vi "about_v1.0.vi"() -> ()   [LabVIEW 2025]
doc: "Use this template to build a producer/consumer design pattern with events to produce queue items. Use this design pattern instead of the User Interface Event Handler pattern for user interfaces when you want to execute code asynchronously in response to an event without slowing the user interface responsiveness."
uses:
  controls/hyperlink.ctl
  controls/linkedin.ctl
  controls/fb.ctl
  controls/youtube.ctl
  controls/insta.ctl
  controls/x.ctl
  <vilib>/Platform/browser.llb/Open URL in Default Browser (string).vi
panel:
  in  "x":T1
  in  "insta":T2
  in  "youtube":T3
  in  "facebook":T4
  in  "linkedin":T5
  in  "producer_exit":bool
  in  "hyperlink":T6
  # "Fresh was founded in 2007 with the vision of pairing design and technology to drive innovation in the emerging digital economy.\n\nJeff Dance and Steve Hulet, our co-founders, imagined multi-disciplinary teams coming together to solve challenges for today and tomorrow, leveraging the best talent and technology in the process.\n\nAs Fresh grows, we remain committed to integrated teams, truly collaborative teamwork, and honing the combination of creative and technical consulting."
  # "Contact Us"
  # "HQ"
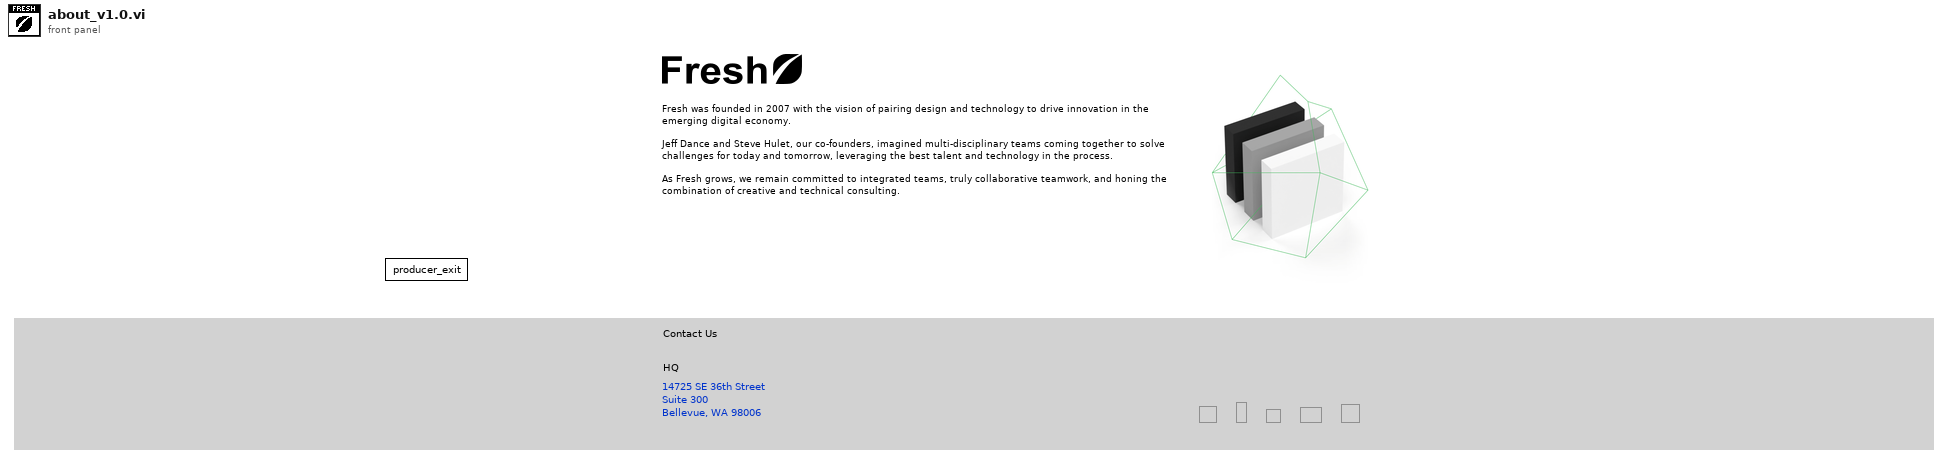
[diagram p1: front panel]
types:
  T1 = typedef "x.ctl" = bool
  T2 = typedef "insta.ctl" = bool
  T3 = typedef "youtube.ctl" = bool
  T4 = typedef "fb.ctl" = bool
  T5 = typedef "linkedin.ctl" = bool
  T6 = typedef "hyperlink.ctl" = bool
  T7 = enum32{"Invalid", "Standard", "Closed", "Hidden", "Minimized", "Maximized"}
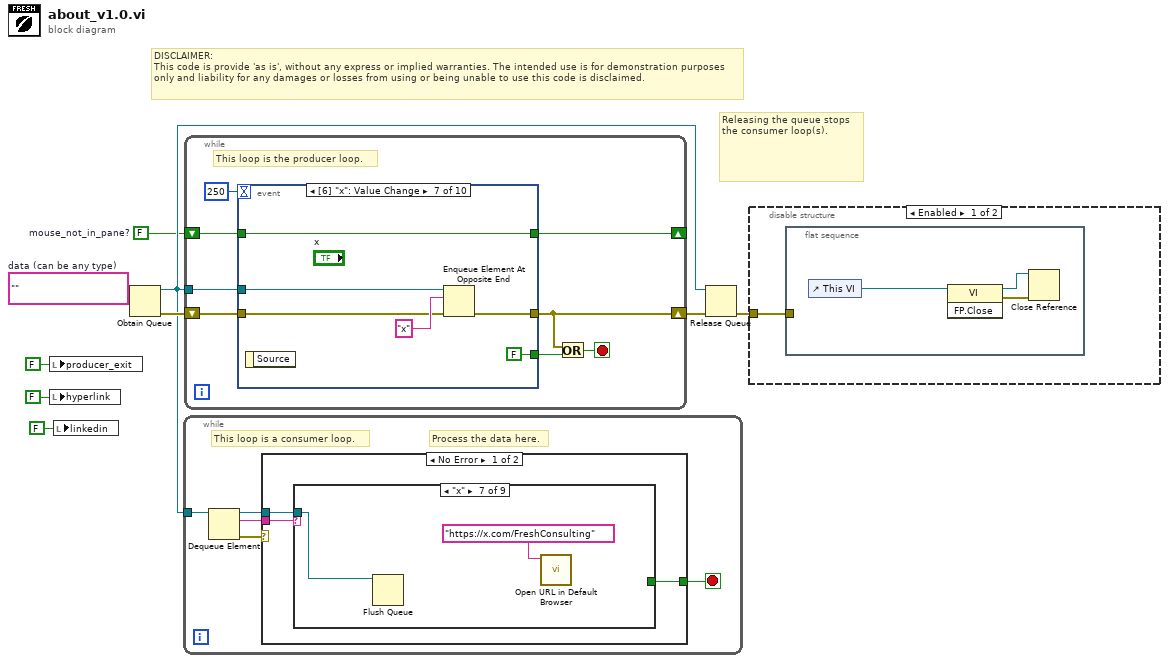
[diagram p0: block diagram]
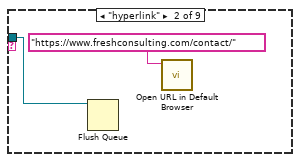
[diagram p4: hidden frame]
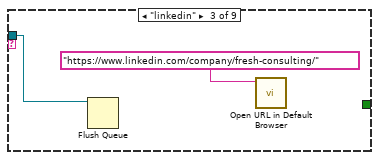
[diagram p5: hidden frame]
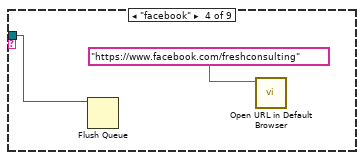
[diagram p6: hidden frame]
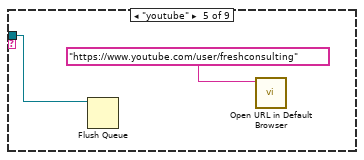
[diagram p7: hidden frame]
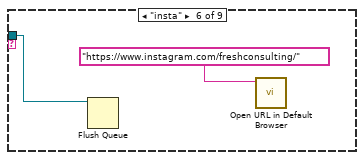
[diagram p8: hidden frame]
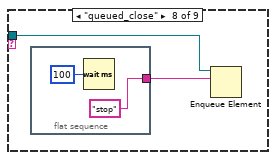
[diagram p9: hidden frame]
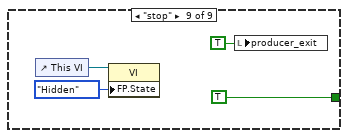
[diagram p10: hidden frame]
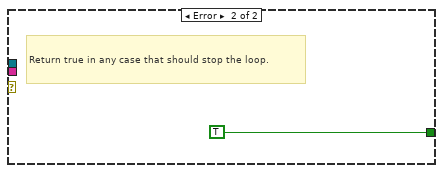
[diagram p11: hidden frame]
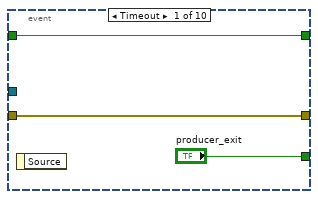
[diagram p12: hidden frame]
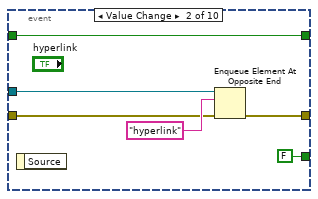
[diagram p13: hidden frame]
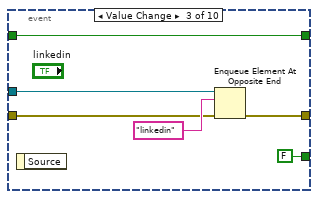
[diagram p14: hidden frame]
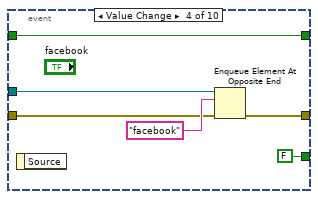
[diagram p15: hidden frame]
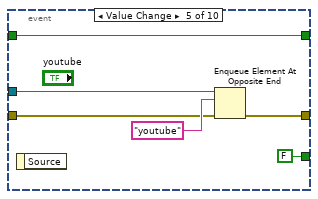
[diagram p16: hidden frame]
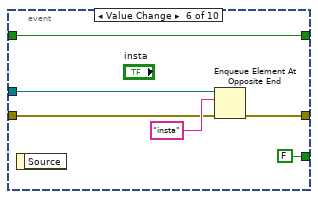
[diagram p17: hidden frame]
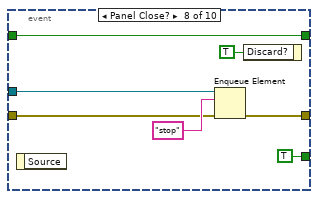
[diagram p18: hidden frame]
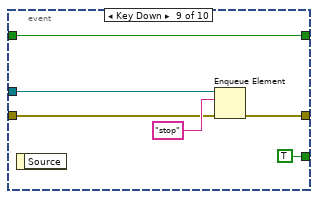
[diagram p19: hidden frame]
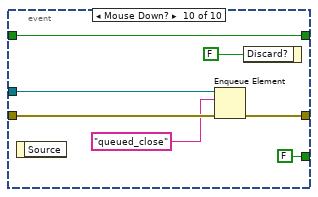
[diagram p20: hidden frame]
diagram:
  w4 = FALSE  # mouse_not_in_pane?
  w7 = ""  # data (can be any type)
  # "DISCLAIMER:\nThis code is provide 'as is', without any express or implied warranties. The intended use is for demonstration purposes only and liability for any damages or losses from using or being unable to use this code is disclaimed."
  # "Releasing the queue stops the consumer loop(s)."
  n1 = local write "producer_exit"(FALSE ("producer_exit")) -> ()
  n2 = local write "hyperlink"(T6 FALSE ("hyperlink")) -> ()
  n3 = local write "linkedin"(T5 FALSE ("linkedin")) -> ()
  n4 = Obtain Queue(element data type=w7) -> (queue out=w6:refnum<queue>, error out=w9:errorcluster)  [unwired: 4 in, 1 out]
  n5 = while {
    tunnel: w6 -> [w14]
    stop <- w11 stop-if-true
    # "Process the data here."
    # "This loop is a consumer loop."
    n6 = Dequeue Element(queue=w14) -> (queue out=w10:refnum<queue>, element=w12:string, error out=w13:errorcluster)  [unwired: 2 in, 1 out]
    n7 = case shown="No Error" w13 {
      tunnel: w12 -> [w17 _]
      tunnel: [w16 TRUE] -> w11
      tunnel: w10 -> [w15 _]
      frame No Error {
        n8 = case shown="\"x\"" w17 {
          tunnel: [_ _ _ _ _ _ _ _ TRUE] -> w16
          tunnel: w15 -> [_ w18 w20 w22 w24 w26 w28 w31 _]
          frame Default {
          }
          frame "hyperlink" {
            n9 = Flush Queue(queue=w18) -> ()  [unwired: 1 in, 3 out]
            n10 = call-poly <vilib>:"Open URL in Default Browser.vi"("URL"="https://www.freshconsulting.com/contact/") -> ()  [unwired: 5 in, 2 out]
          }
          frame "linkedin" {
            n11 = Flush Queue(queue=w20) -> ()  [unwired: 1 in, 3 out]
            n12 = call-poly <vilib>:"Open URL in Default Browser.vi"("URL"="https://www.linkedin.com/company/fresh-consulting/") -> ()  [unwired: 5 in, 2 out]
          }
          frame "facebook" {
            n13 = Flush Queue(queue=w22) -> ()  [unwired: 1 in, 3 out]
            n14 = call-poly <vilib>:"Open URL in Default Browser.vi"("URL"="https://www.facebook.com/freshconsulting") -> ()  [unwired: 5 in, 2 out]
          }
          frame "youtube" {
            n15 = Flush Queue(queue=w24) -> ()  [unwired: 1 in, 3 out]
            n16 = call-poly <vilib>:"Open URL in Default Browser.vi"("URL"="https://www.youtube.com/user/freshconsulting") -> ()  [unwired: 5 in, 2 out]
          }
          frame "insta" {
            n17 = Flush Queue(queue=w26) -> ()  [unwired: 1 in, 3 out]
            n18 = call-poly <vilib>:"Open URL in Default Browser.vi"("URL"="https://www.instagram.com/freshconsulting/") -> ()  [unwired: 5 in, 2 out]
          }
          frame "x" {
            n19 = Flush Queue(queue=w28) -> ()  [unwired: 1 in, 3 out]
            n20 = call-poly <vilib>:"Open URL in Default Browser.vi"("URL"="https://x.com/FreshConsulting") -> ()  [unwired: 5 in, 2 out]
          }
          frame "queued_close" {
            n21 = flat-sequence {
              tunnel: ["stop" ("element")] -> w30
              frame #0 {
                n22 = Wait (ms)(milliseconds to wait=u32 100) -> ()  [unwired: 1 out]
              }
            }
            n23 = Enqueue Element(queue=w31, element=w30) -> ()  [unwired: 2 in, 3 out]
          }
          frame "stop" {
            n24 = control-ref of="This VI"() -> (w34:refnum<vi>)
            n25 = property class="VI"(reference=w34, "FP.State"=T7."Hidden" ("Front Panel Window:State")) -> ()  [unwired: 1 in, 2 out]
            n26 = local write "producer_exit"(TRUE ("producer_exit")) -> ()
          }
        }
      }
      frame Error {
        # "Return true in any case that should stop the loop."
      }
    }
  }
  n27 = while {
    shift-right: [w42] -> w8
    shift-left: w9 -> [w45]
    tunnel: w6 -> [w46]
    shift-right: [w40] -> _
    shift-left: w4 -> [w41]
    stop <- w43 stop-if-true
    # "This loop is the producer loop."
    n28 = event shown="[6] \"x\": Value Change" {
      selector: _ -> [_ _ _ _ _ _ _ _ _ _]
      dyn-events: _ -> [_ _ _ _ _ _ _ _ _ _]
      timeout: 250 -> [_ _ _ _ _ _ _ _ _ _]
      tunnel: w46 -> [_ w54 w60 w66 w72 w78 w84 w91 w97 w105]
      tunnel: w45 -> [w48 w53 w59 w65 w71 w77 w83 w90 w96 w104]
      tunnel: [w48 w52 w58 w64 w70 w76 w82 w89 w95 w103] -> w42
      tunnel: ["producer_exit" FALSE ("stop") FALSE ("stop") FALSE ("stop") FALSE ("stop") FALSE ("stop") FALSE ("stop") TRUE ("stop") TRUE ("stop") FALSE ("stop")] -> w44
      tunnel: w41 -> [w49 w50 w56 w62 w68 w74 w80 w86 w93 w101]
      tunnel: [w49 w50 w56 w62 w68 w74 w80 w86 w93 w101] -> w40
      event Timeout {
        n29 = event-data() -> ()  [unwired: 1 in, 1 out]
      }
      event Value Change {
        n30 = event-data() -> ()  [unwired: 1 in, 1 out]
        n31 = Enqueue Element At Opposite End(queue=w54, element="hyperlink", error in (no error)=w53) -> (error out=w52:errorcluster)  [unwired: 1 in, 2 out]
      }
      event Value Change {
        n32 = event-data() -> ()  [unwired: 1 in, 1 out]
        n33 = Enqueue Element At Opposite End(queue=w60, element="linkedin", error in (no error)=w59) -> (error out=w58:errorcluster)  [unwired: 1 in, 2 out]
      }
      event Value Change {
        n34 = event-data() -> ()  [unwired: 1 in, 1 out]
        n35 = Enqueue Element At Opposite End(queue=w66, element="facebook", error in (no error)=w65) -> (error out=w64:errorcluster)  [unwired: 1 in, 2 out]
      }
      event Value Change {
        n36 = event-data() -> ()  [unwired: 1 in, 1 out]
        n37 = Enqueue Element At Opposite End(queue=w72, element="youtube", error in (no error)=w71) -> (error out=w70:errorcluster)  [unwired: 1 in, 2 out]
      }
      event Value Change {
        n38 = event-data() -> ()  [unwired: 1 in, 1 out]
        n39 = Enqueue Element At Opposite End(queue=w78, element="insta", error in (no error)=w77) -> (error out=w76:errorcluster)  [unwired: 1 in, 2 out]
      }
      event Value Change {
        n40 = event-data() -> ()  [unwired: 1 in, 1 out]
        n41 = Enqueue Element At Opposite End(queue=w84, element="x", error in (no error)=w83) -> (error out=w82:errorcluster)  [unwired: 1 in, 2 out]
      }
      event Panel Close? {
        n42 = event-data() -> ()  [unwired: 1 in, 1 out]
        n43 = Enqueue Element(queue=w91, element="stop", error in (no error)=w90) -> (error out=w89:errorcluster)  [unwired: 1 in, 2 out]
        n44 = event-data("Discard?"=TRUE) -> ()  [unwired: 1 in, 1 out]
      }
      event Key Down {
        n45 = event-data() -> ()  [unwired: 1 in, 1 out]
        n46 = Enqueue Element(queue=w97, element="stop", error in (no error)=w96) -> (error out=w95:errorcluster)  [unwired: 1 in, 2 out]
      }
      event Mouse Down? {
        n47 = event-data() -> ()  [unwired: 1 in, 1 out]
        n48 = Enqueue Element(queue=w105, element="queued_close", error in (no error)=w104) -> (error out=w103:errorcluster)  [unwired: 1 in, 2 out]
        n49 = event-data("Discard?"=FALSE) -> ()  [unwired: 1 in, 1 out]
      }
    }
    n50 = Or(x=w42, y=w44) -> (x .or. y?=w43:bool)
  }
  n51 = Release Queue(queue=w6, error in (no error)=w8) -> (error out=w5:errorcluster)  [unwired: 1 in, 2 out]
  n52 = disable-structure shown="Enabled" {
    disable-tunnel: w5 -> [w106 _]
    frame Enabled {
      n53 = flat-sequence {
        tunnel: w106 -> [_]
        frame #0 {
          n54 = control-ref of="This VI"() -> (w107:refnum<vi>)
          n55 = invoke class="VI" method="FP.Close"(reference=w107) -> (reference out=w108:refnum<vi>, error out=w109:errorcluster)  [unwired: 2 in, 1 out]
          n56 = Close Reference(reference=w108, error in (no error)=w109) -> ()  [unwired: 1 out]
        }
      }
    }
    frame Disabled {
    }
  }
